vi "3_2.vi"() -> ()   [LabVIEW 2023]
uses:
  Misc/InputEnum.ctl
  <vilib>/Utility/miscctls.llb/LVMapReplaceAction.ctl
panel:
  in  "Input Type":T1
  out "x*y 2":i32
  out "Formatted 1D String Array":string[](array[string])
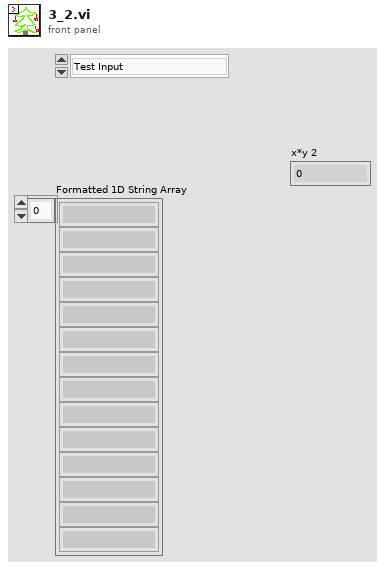
[diagram p1: front panel]
types:
  T1 = typedef "InputEnum.ctl" = enum16{"Test Input", "Real Input"}
  T2 = typedef "LVMapReplaceAction.ctl" = enum32{"Modify Entry only if found", "Add or Modify Entry", "Delete Entry"}
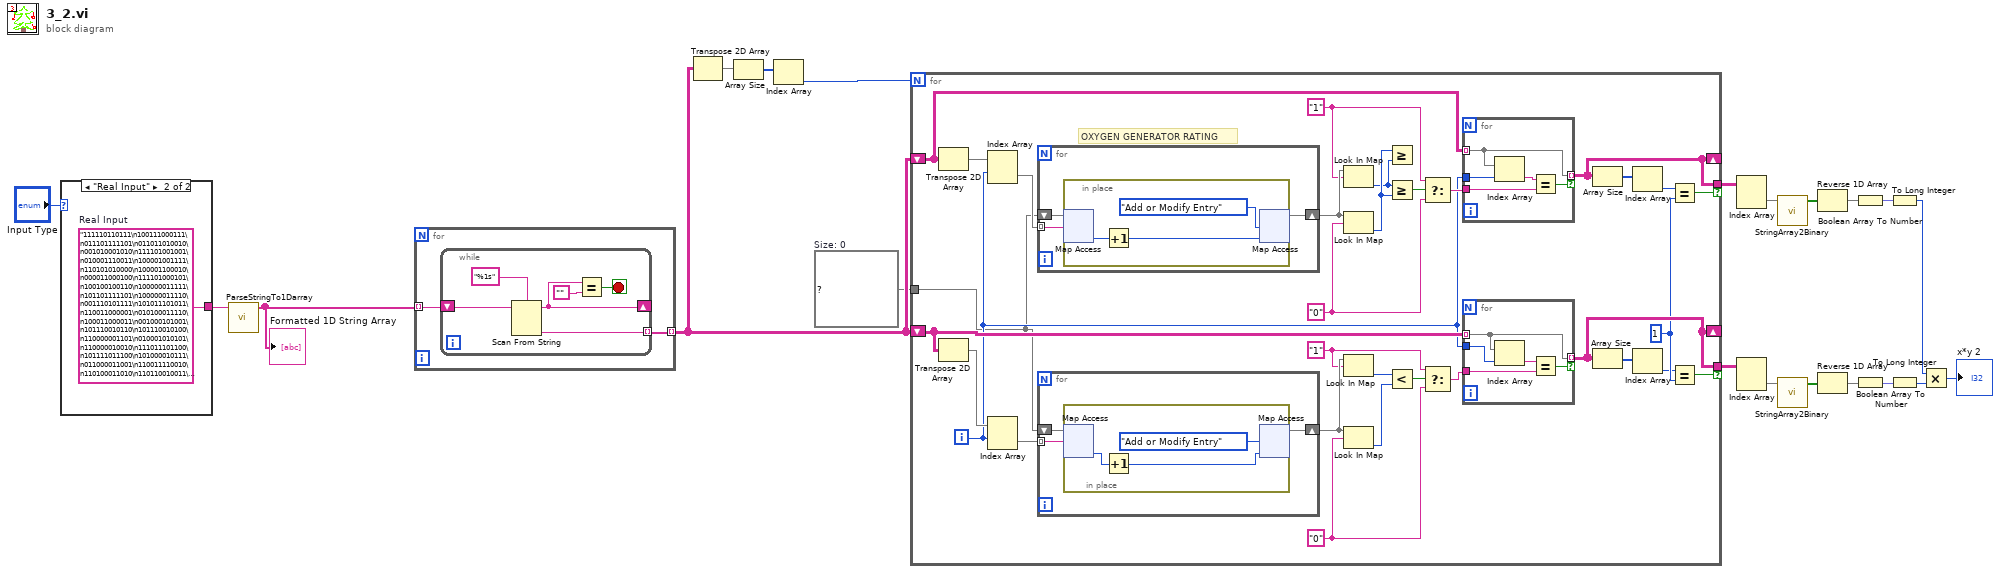
[diagram p0: block diagram]
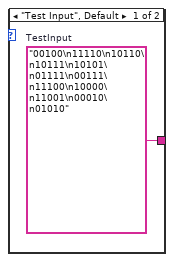
[diagram p2: hidden frame]
diagram:
  w1 = map{string, i32} {}  # Size: 0
  n1 = case shown="\"Real Input\"" "Input Type" {
    tunnel: [w22 w23] -> w3
    frame "Test Input", Default {
      w22 = "00100\n11110\n10110\n10111\n10101\n01111\n00111\n11100\n10000\n11001\n00010\n01010"  # TestInput
    }
    frame "Real Input" {
      w23 = "111110110111\n100111000111\n011101111101\n011011010010\n001010001010\n111101001001\n010001110011\n100001001111\n110101010000\n100001100010\n000011000100\n111101000101\n100100100110\n100000011111\n101101111101\n100000011110\n001110101111\n101011101011\n110011000001\n010100011110\n100011000011\n001000101001\n101110010110\n101110010100\n110000001101\n010001010101\n110000010010\n111011101100\n101111011100\n101000010111\n011000011001\n110011110010\n110100011010\n110110010011\n001110001100\n011011001100\n000011101111\n111010101001\n000101001000\n000010111111\n110100100111\n011000101000\n101011001101\n000110110110\n010101001111\n010011010110\n10..."  # Real Input
    }
  }
  n2 = call "ParseStringTo1Darray.vi"("Copied Input From Advent Of Code Website"=w3) -> ("Formatted 1D String Array"=w21:string[])  [unwired: 10 in]
  "Formatted 1D String Array" <- w21
  n3 = for {
    tunnel: w21 -> [w25] mode=indexing
    tunnel: [w24] -> w20 mode=indexing
    n4 = while {
      shift-right: [w28] -> _
      shift-left: w25 -> [w26]
      tunnel: [w27] -> w24 mode=indexing
      stop <- w29 stop-if-true
      n5 = Scan From String(format string="%1s", input string=w26) -> (remaining string=w28:string, output 1=w27:string)  [unwired: 3 in, 2 out]
      n6 = Equal?(x=w28, y="") -> (x = y?=w29:bool)
    }
  }
  n7 = Transpose 2D Array(2D array=w20) -> (transposed array=w19:string[][])
  n8 = Array Size(array=w19) -> (size(s)=w18:i32[])
  n9 = Index Array(array=w18) -> (element=w17:i32)  [unwired: 1 in]
  n10 = for {
    N: w17 -> [_]
    shift-right: [w53] -> _
    shift-left: w20 -> [w51]
    shift-right: [w41] -> _
    shift-left: w20 -> [w48]
    tunnel: [w53] -> w16 if=w52
    tunnel: [w41] -> w15 if=w40
    tunnel: w1 -> [w32]
    i -> [w46]
    w33 = "0" ("key")
    w36 = "1" ("key")
    w39 = 1 ("y")
    w57 = "0" ("key")
    w56 = "1" ("key")
    # "OXYGEN GENERATOR RATING"
    n11 = Transpose 2D Array(2D array=w51) -> (transposed array=w49:string[][])
    n12 = Transpose 2D Array(2D array=w48) -> (transposed array=w47:string[][])
    n13 = Index Array(array=w49, index (row)=w46) -> (element=w50:string[])  [unwired: 1 in]
    n14 = Index Array(array=w47, index (row)=w46) -> (element=w45:string[])  [unwired: 1 in]
    n15 = for {
      tunnel: w50 -> [w75] mode=indexing
      shift-right: [w74] -> w62
      shift-left: w32 -> [w76]
      n16 = in-place {
        n17 = in-place-map #1(w76, w75) -> (w79:i32)  [unwired: 1 in, 1 out]
        n18 = Increment(x=w79) -> (x+1=w78:i32)
        n19 = in-place-map #1(w78, LVMapReplaceAction."Add or Modify Entry" ("action")) -> (w74:map{string, i32})  [unwired: 2 out]
      }
    }
    n20 = for {
      tunnel: w45 -> [w64] mode=indexing
      shift-right: [w63] -> w44
      shift-left: w32 -> [w65]
      n21 = in-place {
        n22 = in-place-map #2(w65, w64) -> (w68:i32)  [unwired: 1 in, 1 out]
        n23 = Increment(x=w68) -> (x+1=w67:i32)
        n24 = in-place-map #2(w67, LVMapReplaceAction."Add or Modify Entry" ("action")) -> (w63:map{string, i32})  [unwired: 2 out]
      }
    }
    n25 = Look In Map(map=w62, key=w56) -> (value=w58:i32)  [unwired: 1 in, 1 out]
    n26 = Look In Map(map=w62, key=w57) -> (value=w59:i32)  [unwired: 1 in, 1 out]
    n27 = Look In Map(map=w44, key=w36) -> (value=w35:i32)  [unwired: 1 in, 1 out]
    n28 = Look In Map(map=w44, key=w33) -> (value=w34:i32)  [unwired: 1 in, 1 out]
    n29 = Greater Or Equal?(x=w59, y=w58) -> ()  [unwired: 1 out]
    n30 = Greater Or Equal?(x=w58, y=w59) -> (x >= y?=w61:bool)
    n31 = Less?(x=w35, y=w34) -> (x < y?=w37:bool)
    n32 = Select(t=w56, s=w61, f=w57) -> (s? t:f=w60:string)
    n33 = Select(t=w36, s=w37, f=w33) -> (s? t:f=w43:string)
    n34 = for {
      tunnel: w51 -> [w70] mode=indexing
      tunnel: w46 -> [w73]
      tunnel: w60 -> [w71]
      tunnel: [w70] -> w53 mode=indexing if=w69
      n35 = Index Array(array=w70, index=w73) -> (element=w72:string)
      n36 = Equal?(x=w72, y=w71) -> (x = y?=w69:bool)
    }
    n37 = for {
      tunnel: w48 -> [w82] mode=indexing
      tunnel: w46 -> [w84]
      tunnel: [w82] -> w41 mode=indexing if=w81
      tunnel: w43 -> [w80]
      n38 = Index Array(array=w82, index=w84) -> (element=w83:string)
      n39 = Equal?(x=w83, y=w80) -> (x = y?=w81:bool)
    }
    n40 = Array Size(array=w53) -> (size(s)=w55:i32[])
    n41 = Array Size(array=w41) -> (size(s)=w42:i32[])
    n42 = Index Array(array=w55) -> (element=w54:i32)  [unwired: 1 in]
    n43 = Index Array(array=w42) -> (element=w38:i32)  [unwired: 1 in]
    n44 = Equal?(x=w54, y=w39) -> (x = y?=w52:bool)
    n45 = Equal?(x=w38, y=w39) -> (x = y?=w40:bool)
  }
  n46 = Index Array(array=w16) -> (element=w14:string[])  [unwired: 2 in]
  n47 = Index Array(array=w15) -> (element=w13:string[])  [unwired: 2 in]
  n48 = call "StringArray2Binary.vi"("Array in"=w14) -> ("Array out"=w12:bool[])  [unwired: 4 in]
  n49 = call "StringArray2Binary.vi"("Array in"=w13) -> ("Array out"=w11:bool[])  [unwired: 4 in]
  n50 = Reverse 1D Array(array=w12) -> (reversed array=w10:bool[])
  n51 = Reverse 1D Array(array=w11) -> (reversed array=w9:bool[])
  n52 = Boolean Array To Number(Boolean array=w10) -> (number=w5:fxp<+,12,12>)
  n53 = Boolean Array To Number(Boolean array=w9) -> (number=w4:fxp<+,12,12>)
  n54 = To Long Integer(number=w5) -> (32bit integer=w6:i32)
  n55 = To Long Integer(number=w4) -> (32bit integer=w7:i32)
  n56 = Multiply(x=w6, y=w7) -> (x*y=→"x*y 2":i32)
